vi "tsc--Color Picker.vi"(6 "VI Position":cluster{"Left":i16, "Top":i16}={"Left"=-1, "Top"=-1}, 11 "input":u32(colorbox)) -> (2 "accepted?":bool, 3 "Resolved Color":u32(colorbox))   [LabVIEW 2021]
doc: "Allow user to pick a color by slider bar entry for RGB values and/or by HEX code entry. See preview of resolved color before accepting or cancelling.\n\n<b>Code Developed By:</b>\nDaniel Coons\nTechnology Service Corporation\nwww.tsc.com/atcs"
uses:
  <vilib>/Utility/miscctls.llb/LVRectTypeDef.ctl
panel:
  in  "Tab Control":enum32{"rgb", "hsl"}(tab)
  in  "R-number":u8(slide) scale=0.0..255.0
  in  "G-number":u8(slide) scale=0.0..255.0
  in  "B-number":u8(slide) scale=0.0..255.0
  out "R":u32[](array[colorbox])
  out "G":u32[](array[colorbox])
  out "B":u32[](array[colorbox])
  in  "R-selector":u8
  in  "G-selector":u8
  in  "B-selector":u8
  in  "H-number":u16(slide) max=360 scale=0.0..255.0
  in  "S-number":u8(slide) max=100 scale=0.0..100.0
  in  "L-number":u8(slide) max=100 scale=0.0..100.0
  out "S":u32[](array[colorbox])
  out "L":u32[](array[colorbox])
  in  "H-selector":u16 max=360
  in  "S-selector":u8 max=100
  in  "L-selector":u8 max=100
  out "H":u32[](array[colorbox])
  in  "cancel":bool
  in  "ok":bool
  in  "Hex Color":u32 format="%06x"
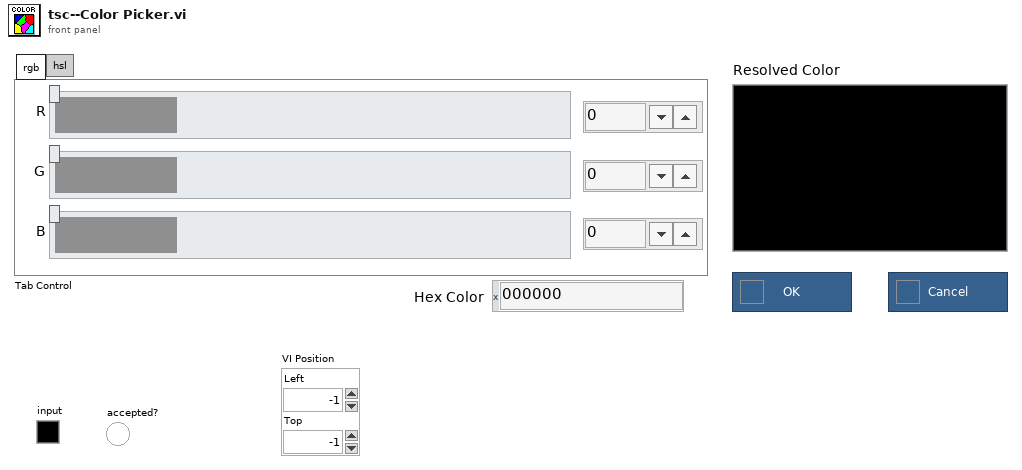
[diagram p1: front panel]
types:
  T1 = typedef "LVRectTypeDef.ctl" = cluster{"Left":i16, "Top":i16, "Right":i16, "Bottom":i16}
  T2 = typedef "LVPointTypeDef.ctl" = cluster{"Horizontal":i16, "Vertical":i16}
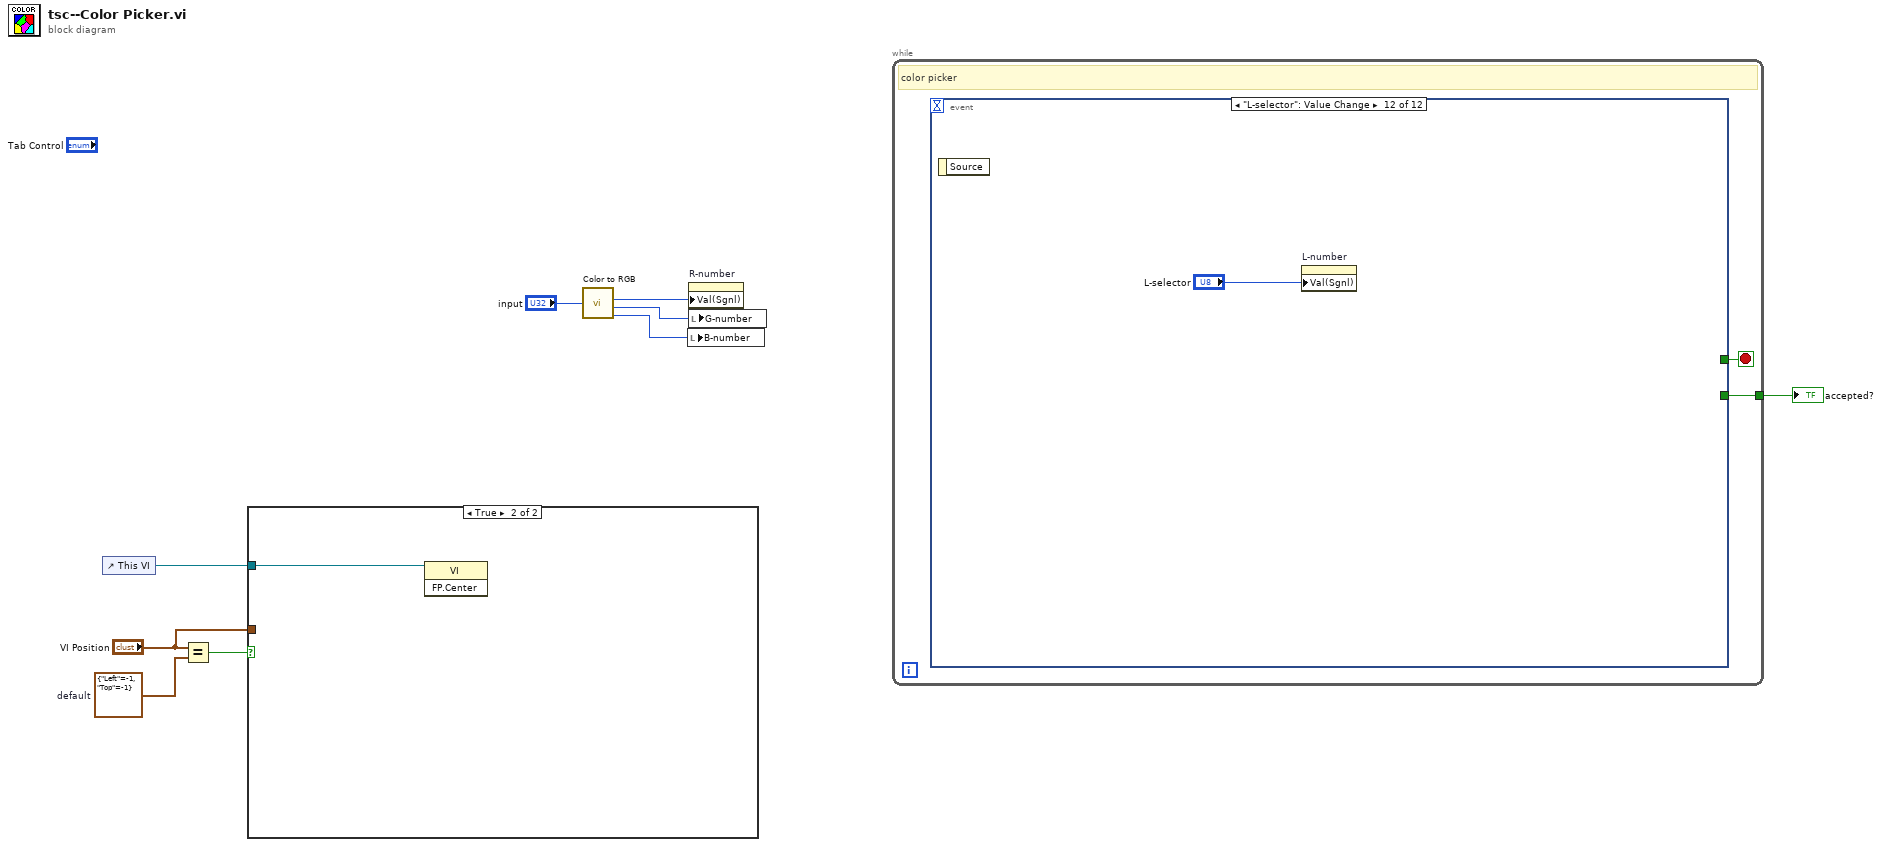
[diagram p0: block diagram]
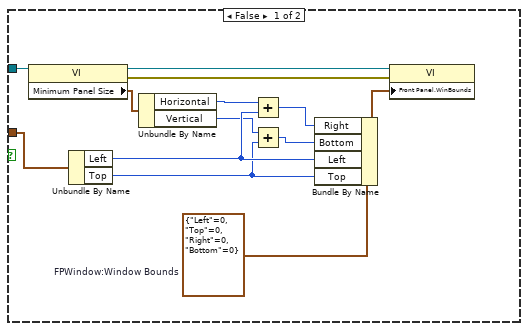
[diagram p2: hidden frame]
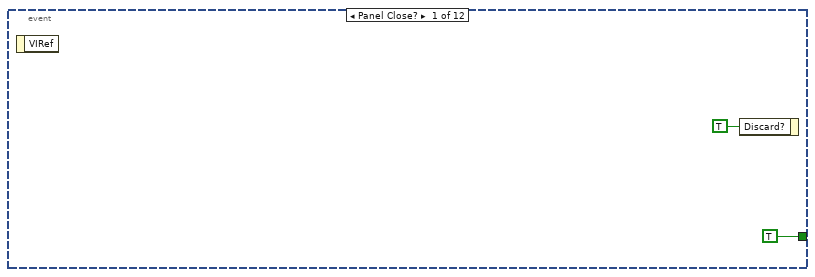
[diagram p3: hidden frame]
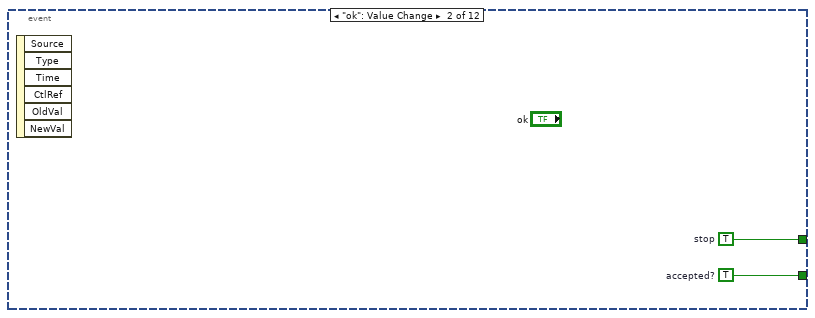
[diagram p4: hidden frame]
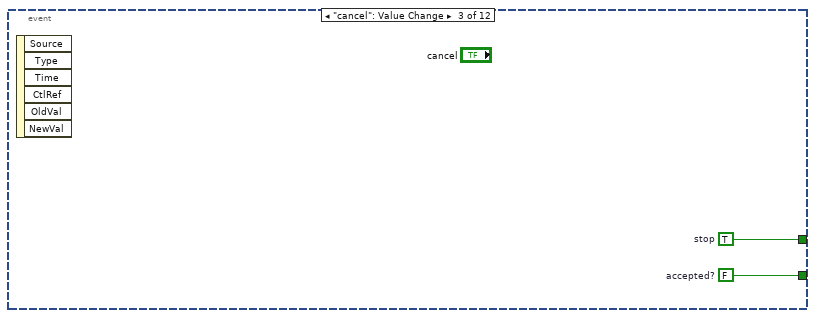
[diagram p5: hidden frame]
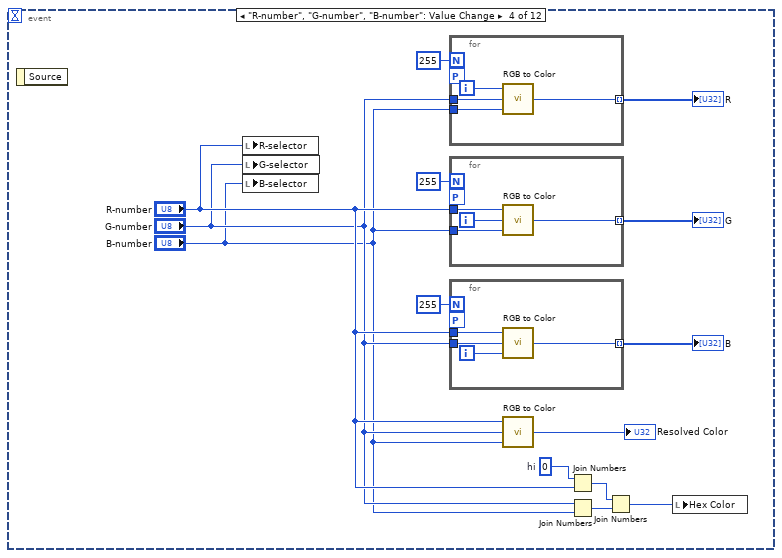
[diagram p6: hidden frame]
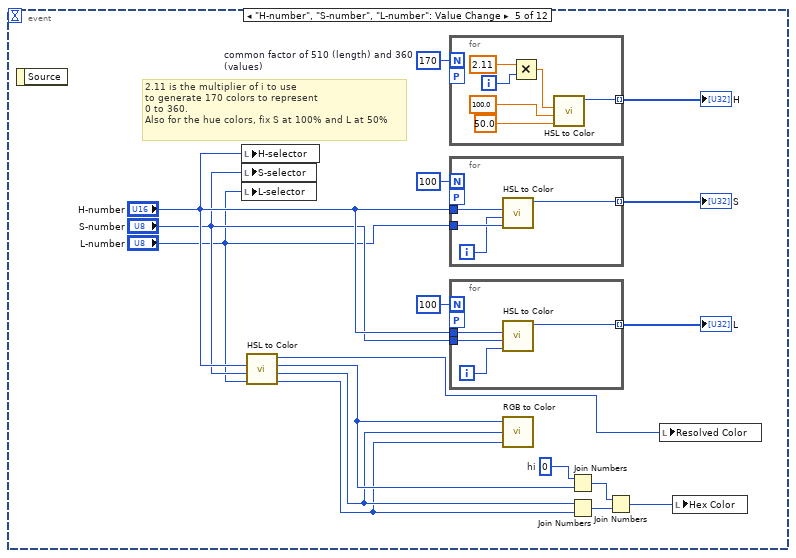
[diagram p7: hidden frame]
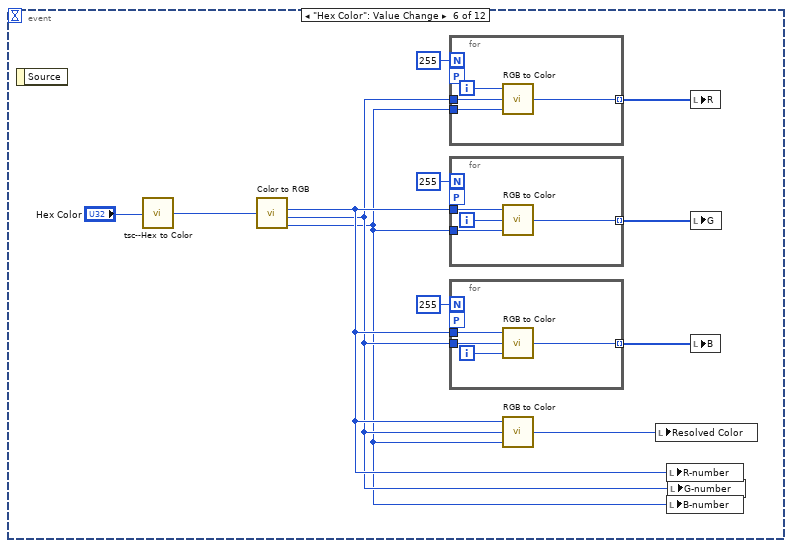
[diagram p8: hidden frame]
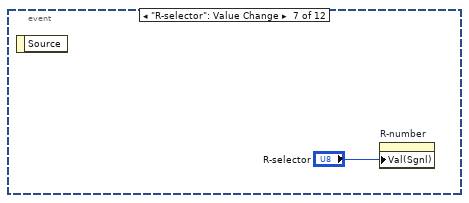
[diagram p9: hidden frame]
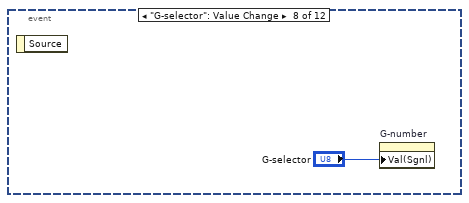
[diagram p10: hidden frame]
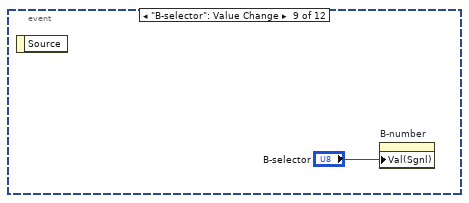
[diagram p11: hidden frame]
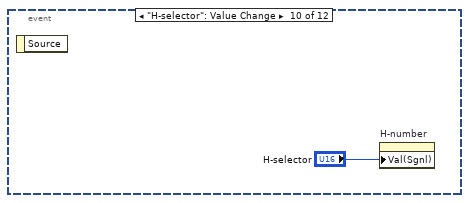
[diagram p12: hidden frame]
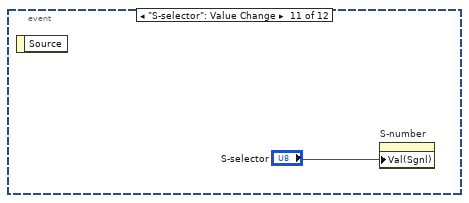
[diagram p13: hidden frame]
diagram:
  w3 = cluster{"Left":i16, "Top":i16} {"Left"=-1, "Top"=-1}  # default
  n1 = control-ref of="This VI"() -> (w4:refnum<vi>)
  n2 = Equal?(x="VI Position", y=w3) -> (x = y?=w2:bool)
  n3 = case shown="True" w2 {
    tunnel: w4 -> [w22 w23]
    tunnel: "VI Position" -> [w18 _]
    frame False {
      w17 = T1 {"Left"=0, "Top"=0, "Right"=0, "Bottom"=0}  # FPWindow:Window Bounds
      n4 = property class="VI"(reference=w22) -> (reference out=w21:refnum<vi>, error out=w20:errorcluster, "Minimum Panel Size"=w19:T2)  [unwired: 1 in]
      n5 = Unbundle By Name(w18) -> ("Left"=w16:i16, "Top"=w11:i16)
      n6 = Unbundle By Name(w19) -> ("Horizontal"=w15:i16, "Vertical"=w12:i16)
      n7 = Add(x=w15, y=w16) -> (x+y=w14:i16)
      n8 = Add(x=w12, y=w11) -> (x+y=w10:i16)
      n9 = Bundle By Name(cluster=w17, "Right"=w14, "Bottom"=w10, "Left"=w16, "Top"=w11) -> (w13:T1)
      n10 = property class="VI"(reference=w21, error in=w20, "Front Panel.WinBounds"=w13) -> ()  [unwired: 2 out]
    }
    frame True {
      n11 = invoke class="VI" method="FP.Center"(reference=w23) -> ()  [unwired: 2 in, 3 out]
    }
  }
  n12 = call <vilib>:"Color to RGB.vi"("Color"="input") -> ("R"=w8:u8, "G"=w7:u8, "B"=w6:u8)  [unwired: 1 out]
  n13 = local write "B-number"(w6) -> ()
  n14 = property on="R-number" class="Slide (strict)"("Val(Sgnl)"=w8) -> ()  [unwired: 2 in, 2 out]
  n15 = local write "G-number"(w7) -> ()
  n16 = while {
    tunnel: [w24] -> w5
    stop <- w25 stop-if-true
    # "color picker"
    n17 = event shown="[11] \"L-selector\": Value Change" {
      selector: _ -> [_ _ _ _ _ _ _ _ _ _ _ _]
      dyn-events: _ -> [_ _ _ _ _ _ _ _ _ _ _ _]
      timeout: _ -> [_ _ _ _ _ _ _ _ _ _ _ _]
      tunnel: [TRUE w29 w31 _ _ _ _ _ _ _ _ _] -> w25
      tunnel: [_ w28 w30 _ _ _ _ _ _ _ _ _] -> w24
      event Panel Close? {
        n18 = event-data() -> ()  [unwired: 1 in, 1 out]
        n19 = event-data("Discard?"=TRUE) -> ()  [unwired: 1 in, 1 out]
      }
      event "ok": Value Change {
        w28 = TRUE  # accepted?
        w29 = TRUE  # stop
        n20 = event-data() -> ()  [unwired: 1 in, 6 out]
      }
      event "cancel": Value Change {
        w30 = FALSE  # accepted?
        w31 = TRUE  # stop
        n21 = event-data() -> ()  [unwired: 1 in, 6 out]
      }
      event "R-number", "G-number", "B-number": Value Change {
        w39 = u8 0  # hi
        n22 = event-data() -> ()  [unwired: 1 in, 1 out]
        n23 = local write "R-selector"("R-number") -> ()
        n24 = local write "G-selector"("G-number") -> ()
        n25 = local write "B-selector"("B-number") -> ()
        n26 = for {
          N: 255 -> [_]
          tunnel: "G-number" -> [w57]
          tunnel: "B-number" -> [w56]
          tunnel: [w54] -> w44 mode=indexing
          workers-P: _ -> [_]
          i -> [w55]
          n27 = call <vilib>:"RGB to Color.vi"("B"=w56, "G"=w57, "R"=w55) -> ("Color"=w54:u32)
        }
        "R" <- w44
        n28 = for {
          N: 255 -> [_]
          tunnel: "B-number" -> [w53]
          tunnel: [w52] -> w41 mode=indexing
          tunnel: "R-number" -> [w50]
          workers-P: _ -> [_]
          i -> [w51]
          n29 = call <vilib>:"RGB to Color.vi"("B"=w53, "G"=w51, "R"=w50) -> ("Color"=w52:u32)
        }
        "G" <- w41
        n30 = for {
          N: 255 -> [_]
          tunnel: "R-number" -> [w47]
          tunnel: [w49] -> w40 mode=indexing
          tunnel: "G-number" -> [w46]
          workers-P: _ -> [_]
          i -> [w48]
          n31 = call <vilib>:"RGB to Color.vi"("B"=w48, "G"=w46, "R"=w47) -> ("Color"=w49:u32)
        }
        "B" <- w40
        n32 = call <vilib>:"RGB to Color.vi"("B"="B-number", "G"="G-number", "R"="R-number") -> ("Color"=→"Resolved Color":u32)
        n33 = Join Numbers(hi=w39, lo="R-number") -> ((hi.lo)=w37:u16)
        n34 = Join Numbers(hi="G-number", lo="B-number") -> ((hi.lo)=w38:u16)
        n35 = Join Numbers(hi=w37, lo=w38) -> ((hi.lo)=w36:u32)
        n36 = local write "Hex Color"(w36) -> ()
      }
      event "H-number", "S-number", "L-number": Value Change {
        w71 = u8 0  # hi
        w74 = 170  # common factor of 510 (length) and 360 (values)
        # "2.11 is the multiplier of i to use\nto generate 170 colors to represent\n0 to 360. \nAlso for the hue colors, fix S at 100% and L at 50%"
        n37 = event-data() -> ()  [unwired: 1 in, 1 out]
        n38 = local write "H-selector"("H-number") -> ()
        n39 = local write "S-selector"("S-number") -> ()
        n40 = local write "L-selector"("L-number") -> ()
        n41 = call "HSL to Color.vi"("L (%)"="L-number", "S (%)"="S-number", "H (degrees)"="H-number") -> ("B"=w59:u8, "G"=w61:u8, "R"=w63:u8, "Color out"=w58:u32)  [unwired: 5 in]
        n42 = for {
          N: w74 -> [_]
          tunnel: [w88] -> w67 mode=indexing
          workers-P: _ -> [_]
          i -> [w84]
          n43 = Multiply(x=2.11, y=w84) -> (x*y=w83:dbl)
          n44 = call "HSL to Color.vi"("L (%)"=50.0, "S (%)"=100.0, "H (degrees)"=w83) -> ("Color out"=w88:u32)  [unwired: 5 in, 3 out]
        }
        "H" <- w67
        n45 = for {
          N: 100 -> [_]
          tunnel: "L-number" -> [w82]
          tunnel: [w81] -> w66 mode=indexing
          tunnel: "H-number" -> [w79]
          workers-P: _ -> [_]
          i -> [w80]
          n46 = call "HSL to Color.vi"("L (%)"=w82, "S (%)"=w80, "H (degrees)"=w79) -> ("Color out"=w81:u32)  [unwired: 5 in, 3 out]
        }
        "S" <- w66
        n47 = for {
          N: 100 -> [_]
          tunnel: "H-number" -> [w76]
          tunnel: [w78] -> w65 mode=indexing
          tunnel: "S-number" -> [w75]
          workers-P: _ -> [_]
          i -> [w77]
          n48 = call "HSL to Color.vi"("L (%)"=w77, "S (%)"=w75, "H (degrees)"=w76) -> ("Color out"=w78:u32)  [unwired: 5 in, 3 out]
        }
        "L" <- w65
        n49 = call <vilib>:"RGB to Color.vi"("B"=w59, "G"=w61, "R"=w63) -> ()  [unwired: 1 out]
        n50 = Join Numbers(hi=w71, lo=w63) -> ((hi.lo)=w69:u16)
        n51 = Join Numbers(hi=w61, lo=w59) -> ((hi.lo)=w70:u16)
        n52 = Join Numbers(hi=w69, lo=w70) -> ((hi.lo)=w68:u32)
        n53 = local write "Resolved Color"(w58) -> ()
        n54 = local write "Hex Color"(w68) -> ()
      }
      event "Hex Color": Value Change {
        n55 = event-data() -> ()  [unwired: 1 in, 1 out]
        n56 = call "tsc--Hex to Color.vi"("Hex String"="Hex Color") -> ("Color"=w96:u32)  [unwired: 4 in]
        n57 = call <vilib>:"Color to RGB.vi"("Color"=w96) -> ("R"=w91:u8, "G"=w90:u8, "B"=w89:u8)  [unwired: 1 out]
        n58 = for {
          N: 255 -> [_]
          tunnel: w90 -> [w112]
          tunnel: w89 -> [w111]
          tunnel: [w109] -> w95 mode=indexing
          workers-P: _ -> [_]
          i -> [w110]
          n59 = call <vilib>:"RGB to Color.vi"("B"=w111, "G"=w112, "R"=w110) -> ("Color"=w109:u32)
        }
        n60 = for {
          N: 255 -> [_]
          tunnel: w89 -> [w108]
          tunnel: [w107] -> w94 mode=indexing
          tunnel: w91 -> [w105]
          workers-P: _ -> [_]
          i -> [w106]
          n61 = call <vilib>:"RGB to Color.vi"("B"=w108, "G"=w106, "R"=w105) -> ("Color"=w107:u32)
        }
        n62 = for {
          N: 255 -> [_]
          tunnel: w91 -> [w102]
          tunnel: [w104] -> w93 mode=indexing
          tunnel: w90 -> [w101]
          workers-P: _ -> [_]
          i -> [w103]
          n63 = call <vilib>:"RGB to Color.vi"("B"=w103, "G"=w101, "R"=w102) -> ("Color"=w104:u32)
        }
        n64 = call <vilib>:"RGB to Color.vi"("B"=w89, "G"=w90, "R"=w91) -> ("Color"=w92:u32)
        n65 = local write "Resolved Color"(w92) -> ()
        n66 = local write "R-number"(w91) -> ()
        n67 = local write "B-number"(w89) -> ()
        n68 = local write "G-number"(w90) -> ()
        n69 = local write "R"(w95) -> ()
        n70 = local write "G"(w94) -> ()
        n71 = local write "B"(w93) -> ()
      }
      event "R-selector": Value Change {
        n72 = event-data() -> ()  [unwired: 1 in, 1 out]
        n73 = property on="R-number" class="Slide (strict)"("Val(Sgnl)"="R-selector") -> ()  [unwired: 2 in, 2 out]
      }
      event "G-selector": Value Change {
        n74 = event-data() -> ()  [unwired: 1 in, 1 out]
        n75 = property on="G-number" class="Slide (strict)"("Val(Sgnl)"="G-selector") -> ()  [unwired: 2 in, 2 out]
      }
      event "B-selector": Value Change {
        n76 = event-data() -> ()  [unwired: 1 in, 1 out]
        n77 = property on="B-number" class="Slide (strict)"("Val(Sgnl)"="B-selector") -> ()  [unwired: 2 in, 2 out]
      }
      event "H-selector": Value Change {
        n78 = event-data() -> ()  [unwired: 1 in, 1 out]
        n79 = property on="H-number" class="Slide (strict)"("Val(Sgnl)"="H-selector") -> ()  [unwired: 2 in, 2 out]
      }
      event "S-selector": Value Change {
        n80 = event-data() -> ()  [unwired: 1 in, 1 out]
        n81 = property on="S-number" class="Slide (strict)"("Val(Sgnl)"="S-selector") -> ()  [unwired: 2 in, 2 out]
      }
      event "L-selector": Value Change {
        n82 = event-data() -> ()  [unwired: 1 in, 1 out]
        n83 = property on="L-number" class="Slide (strict)"("Val(Sgnl)"="L-selector") -> ()  [unwired: 2 in, 2 out]
      }
    }
  }
  "accepted?" <- w5
